vi "median.vi"(4 "State":i16, 5 "Time":dbl format="%.2f", 6 "Sensor Values":dbl[](array[numeric]), 7 "Set Points":dbl[](array[numeric])) -> (0 "required data":T1={"Set Point names"=["update (s)", "samples (N)", "data"], "required number of setpoints"=3, "required number of sensors"=0, "Sensor names"=[]}, 3 "output value":dbl)   [LabVIEW 2019]
uses:
  <vilib>/ptbypt/NI_PtbyPt.lvlib
  <vilib>/Analysis/NI_AALBase.lvlib
panel:
  out "Current Queue":dbl[](array[numeric])
  # "Enter the correct information for this control code in the required data structure below. Then make the current value default by right clicking on the border of the data structure. Select \"data operations\" and then select \"make current value default\". These values will be displayed by process controller."
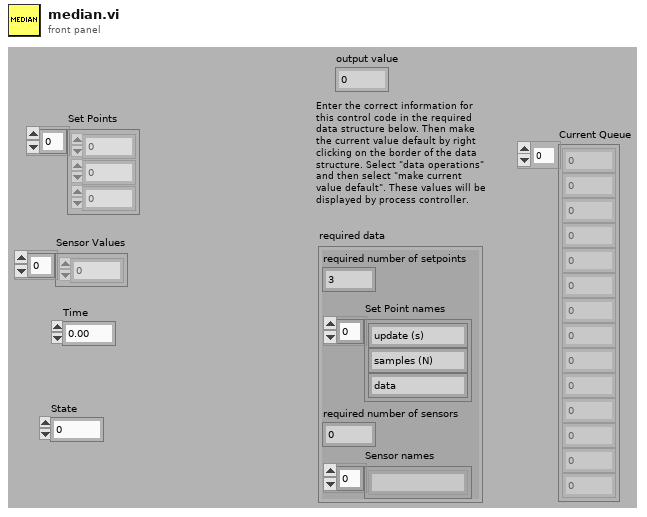
[diagram p1: front panel]
types:
  T1 = cluster{"Set Point names":string[], "required number of setpoints":u8, "required number of sensors":u8, "Sensor names":string[]}
  T2 = cluster{"Set Points[0]":dbl, "Set Points[1]":dbl, "Set Points[2]":dbl}
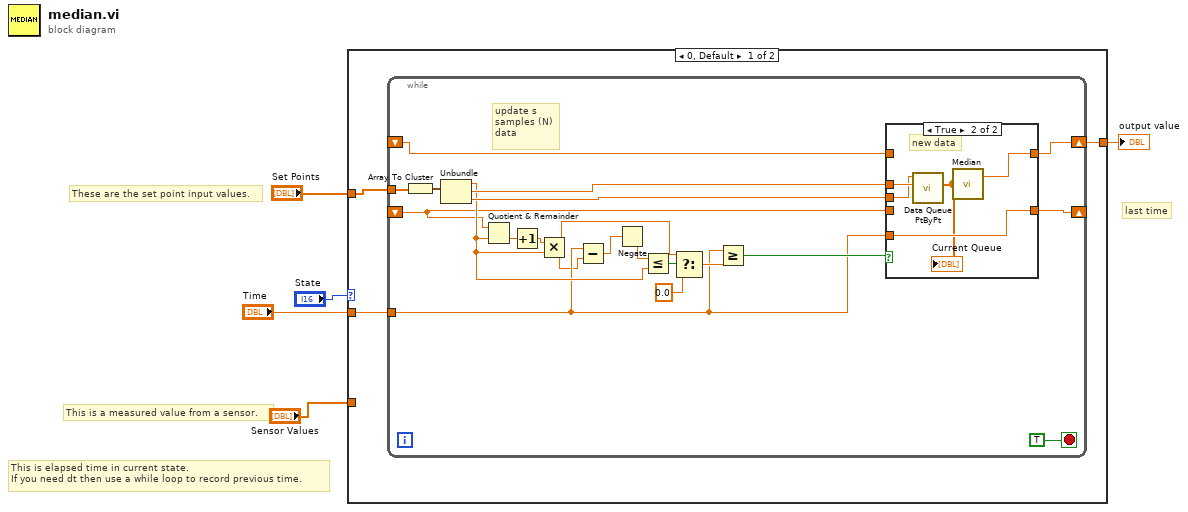
[diagram p0: block diagram]
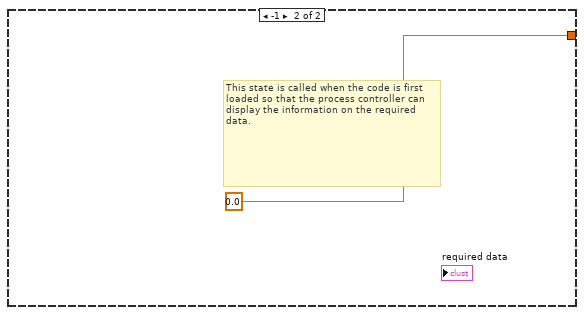
[diagram p3: hidden frame]
diagram:
  # "last time"
  # "These are the set point input values."
  # "This is a measured value from a sensor."
  # "This is elapsed time in current state.\nIf you need dt then use a while loop to record previous time."
  n1 = case shown="0, Default" "State" {
    tunnel: [w6 0.0 ("fraction on")] -> w4
    tunnel: "Set Points" -> [w7 _]
    tunnel: "Sensor Values" -> [_ _]
    tunnel: "Time" -> [w8 _]
    frame 0, Default {
      n2 = while {
        shift-right: [w28] -> _
        shift-left: _ -> [w10]
        tunnel: w8 -> [w12]
        tunnel: w7 -> [w25]
        shift-right: [w20] -> w6
        shift-left: _ -> [w19]
        stop <- TRUE stop-if-true
        # "update s\nsamples (N)\ndata"
        n3 = Array To Cluster(array=w25) -> (cluster=w24:T2)
        n4 = Unbundle(w24) -> ("Set Points[0]"=w16:dbl, "Set Points[1]"=w22:dbl, "Set Points[2]"=w23:dbl)
        n5 = Quotient & Remainder(x=w10, y=w16) -> (floor(x/y)=w27:dbl)  [unwired: 1 out]
        n6 = Increment(x=w27) -> (x+1=w26:dbl)
        n7 = Multiply(x=w26, y=w16) -> (x*y=w9:dbl)
        n8 = Subtract(x=w12, y=w9) -> (x-y=w18:dbl)
        n9 = Negate(x=w18) -> (-x=w17:dbl)
        n10 = Less Or Equal?(x=w17, y=w16) -> (x <= y?=w15:bool)
        n11 = Select(t=w9, s=w15, f=0.0 ("Time")) -> (s? t:f=w14:dbl)
        n12 = Greater Or Equal?(x=w12, y=w14) -> (x >= y?=w13:bool)
        n13 = case shown="True" w13 {
          tunnel: [w30 w35] -> w28
          tunnel: w12 -> [_ w35]
          tunnel: w10 -> [w30 _]
          tunnel: w23 -> [_ w31]
          tunnel: w22 -> [_ w34]
          tunnel: [w29 w32] -> w20
          tunnel: w19 -> [w29 _]
          frame False {
          }
          frame True {
            # "new data"
            n14 = call <vilib>:"Data Queue PtByPt.vi"("sample length"=w34, "input data point"=w31) -> ("Current Queue"=w33:dbl[])  [unwired: 5 in, 4 out]
            "Current Queue" <- w33
            n15 = call <vilib>:"Median.vi"("X"=w33) -> ("median"=w32:dbl)  [unwired: 1 out]
          }
        }
      }
    }
    frame -1 {
      # "This state is called when the code is first loaded so that the process controller can display the information on the required data."
    }
  }
  "output value" <- w4
